vi "Help.vi"(5 "error in":errorcluster) -> (0 "error out":errorcluster)   [LabVIEW 2017]
panel:
  in  "Close":bool
  out "new picture":picture
  # "Marvin Tester Version V1.0.\nDeveloped by Redler Technologies.\nAll Rights Reserved.\nhttps://www.redler.co.il/"
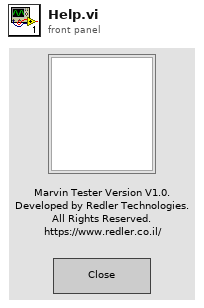
[diagram p1: front panel]
types:
  T1 = typedef "imagedata.ctl" = cluster{"image type":i32, "image depth":i32, "image":u8[], "mask":u8[], "colors":u32[], "Rectangle":cluster{"left":i16, "top":i16, "right":i16, "bottom":i16}}
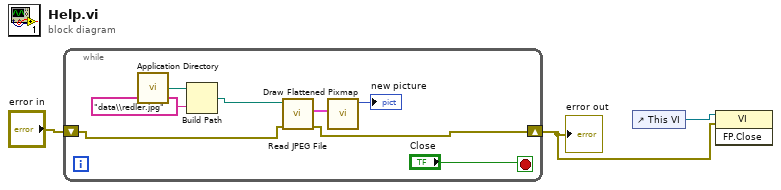
[diagram p0: block diagram]
diagram:
  n1 = while {
    shift-right: [w5] -> w1
    shift-left: "error in" -> [w4]
    stop <- "Close" stop-if-true
    n2 = call <vilib>:"Application Directory.vi"() -> ("Application Directory"=w7:path)
    n3 = Build Path(base path=w7, name or relative path="data\\redler.jpg") -> (appended path=w6:path)
    n4 = call <vilib>:"Read JPEG File.vi"("error in (no error)"=w4, "path to JPEG file"=w6) -> ("error out"=w5:errorcluster, "image data"=w11:T1)  [unwired: 7 in, 1 out]
    n5 = call <vilib>:"Draw Flattened Pixmap.vi"("image data"=w11) -> ("new picture"=→"new picture":picture)  [unwired: 8 in]
  }
  "error out" <- w1
  n6 = control-ref of="This VI"() -> (w2:refnum<vi>)
  n7 = invoke class="VI" method="FP.Close"(reference=w2, error in=w1) -> ()  [unwired: 1 in, 3 out]
